vi "Keithley 2002 DCV Config.vi"(0 "GPIB address":string="16", 1 "range value (volts)":dbl=1000.0 min=0.2 max=1000.0 format="%^.2e", 2 "range (auto:0)":u16(ring) items=["autorange", "autorange once", "set min range", "set max range", "set range value"], 3 "dig. filter count":dbl=10.0 min=1.0 max=100.0 step=1.0 format="%^.2e", 4 "digital filter (off:0)":u16(ring) items=["off", "auto filter", "auto filter once", "moving filter", "repeating filter"], 5 "integration time (0:auto)":u16(ring) items=["automatic", "automatic once", "set to minimum", "set to maximum", "set aperature value", "set NPLC value"], 7 "integ. value":dbl=0.01667 format="%^.2e", 8 "advanced filter (off:0)":u16(ring) items=["off", "enabled"], 9 "resolution (4.5 digits:3)":u16(ring)=3 items=["auto resolution", "auto resolution once", "3.5 digits", "4.5 digits", "5.5 digits", "6.5 digits", "7.5 digits", "8.5 digits"], 10 "noise tolerance (%)":dbl=1.0 min=0.0 max=100.0 step=1.0 format="%^.2e", 11 "error in":T1, 12 "reference (off:0)":u16(ring) items=["off", "set reference value"], 13 "reference value (volts)":dbl min=-1100.0 max=1100.0 format="%^.2e") -> (15 "error out":T1)   [LabVIEW 2020]
doc: "This VI is used to configure the settings for the DC voltage measurements. The instrument can be in any mode when this VI is run. The settings will go into effect and the instrument will go into the DC voltage mode."
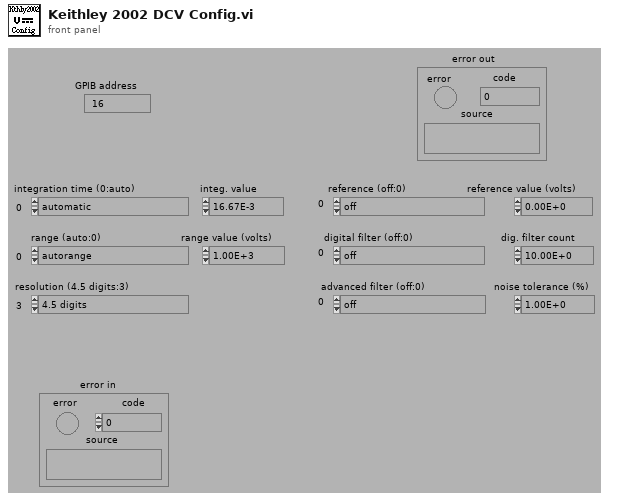
[diagram p1: front panel]
types:
  T1 = cluster{"error":bool, "code":i32, "source":string}
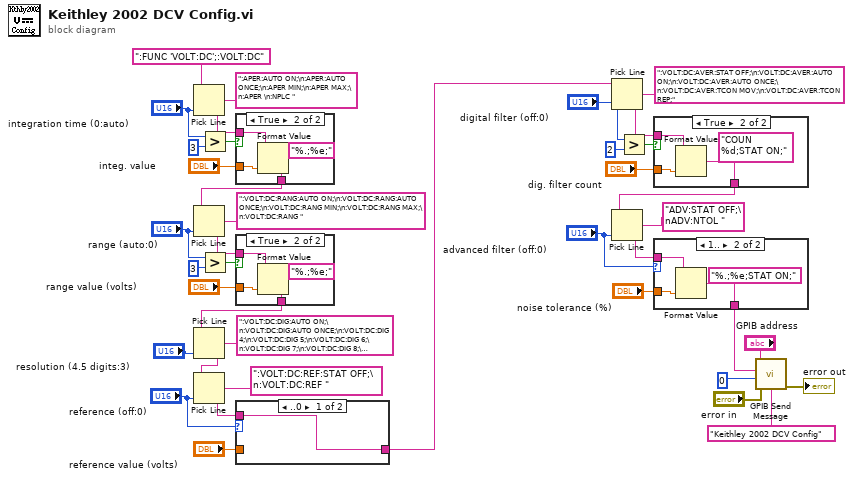
[diagram p0: block diagram]
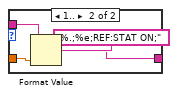
[diagram p4: hidden frame]
diagram:
  n1 = Pick Line(string ("")=":FUNC 'VOLT:DC';:VOLT:DC", multi-line string=":APER:AUTO ON;\n:APER:AUTO ONCE;\n:APER MIN;\n:APER MAX;\n:APER \n:NPLC ", line index="integration time (0:auto)") -> (output string=w34:string)
  n2 = Greater?(x="integration time (0:auto)", y=3) -> (0:w35:bool)
  n3 = Greater?(x="range (auto:0)", y=3) -> (0:w32:bool)
  n4 = case shown="True" w35 {
    tunnel: "integ. value" -> [_ w44]
    tunnel: w34 -> [w41 w43]
    tunnel: [w41 w42] -> w27
    frame False {
    }
    frame True {
      n5 = Format Value(string ("")=w43, format string="%.;%e;", value (0)=w44) -> (output string=w42:string)
    }
  }
  n6 = Pick Line(string ("")=w27, multi-line string=":VOLT:DC:RANG:AUTO ON;\n:VOLT:DC:RANG:AUTO ONCE;\n:VOLT:DC:RANG MIN;\n:VOLT:DC:RANG MAX;\n:VOLT:DC:RANG ", line index="range (auto:0)") -> (output string=w33:string)
  n7 = case shown="True" w32 {
    tunnel: "range value (volts)" -> [_ w49]
    tunnel: w33 -> [w46 w48]
    tunnel: [w46 w47] -> w24
    frame False {
    }
    frame True {
      n8 = Format Value(string ("")=w48, format string="%.;%e;", value (0)=w49) -> (output string=w47:string)
    }
  }
  n9 = Pick Line(string ("")=w24, multi-line string=":VOLT:DC:DIG:AUTO ON;\n:VOLT:DC:DIG:AUTO ONCE;\n:VOLT:DC:DIG 4;\n:VOLT:DC:DIG 5;\n:VOLT:DC:DIG 6;\n:VOLT:DC:DIG 7;\n:VOLT:DC:DIG 8;\n:Volt:DC:Dig 9;", line index="resolution (4.5 digits:3)") -> (output string=w20:string)
  n10 = Pick Line(string ("")=w20, multi-line string=":VOLT:DC:REF:STAT OFF;\n:VOLT:DC:REF ", line index="reference (off:0)") -> (output string=w23:string)
  n11 = case shown="..0" "reference (off:0)" {
    tunnel: "reference value (volts)" -> [_ w55]
    tunnel: w23 -> [w51 w54]
    tunnel: [w51 w52] -> w1
    frame ..0 {
    }
    frame 1.. {
      n12 = Format Value(string ("")=w54, format string="%.;%e;REF:STAT ON;", value (0)=w55) -> (output string=w52:string)
    }
  }
  n13 = Pick Line(string ("")=w1, multi-line string=":VOLT:DC:AVER:STAT OFF;\n:VOLT:DC:AVER:AUTO ON;\n:VOLT:DC:AVER:AUTO ONCE;\n:VOLT:DC:AVER:TCON MOV;\n:VOLT:DC:AVER:TCON REP;", line index="digital filter (off:0)") -> (output string=w17:string)
  n14 = Greater?(x="digital filter (off:0)", y=2) -> (0:w14:bool)
  n15 = case shown="True" w14 {
    tunnel: "dig. filter count" -> [_ w60]
    tunnel: w17 -> [w56 w59]
    tunnel: [w56 w58] -> w6
    frame False {
    }
    frame True {
      n16 = Format Value(string ("")=w59, format string="COUN %d;STAT ON;", value (0)=w60) -> (output string=w58:string)
    }
  }
  n17 = Pick Line(string ("")=w6, multi-line string="ADV:STAT OFF;\nADV:NTOL ", line index="advanced filter (off:0)") -> (output string=w10:string)
  n18 = case shown="1.." "advanced filter (off:0)" {
    tunnel: "noise tolerance (%)" -> [_ w65]
    tunnel: w10 -> [w61 w64]
    tunnel: [w61 w63] -> w7
    frame ..0 {
    }
    frame 1.. {
      n19 = Format Value(string ("")=w64, format string="%.;%e;STAT ON;", value (0)=w65) -> (output string=w63:string)
    }
  }
  n20 = call "GPIB Send Message.vi"("address string"="GPIB address", "write buffer"=w7, "source"="Keithley 2002 DCV Config", "write mode (set END:0)"=0, "error in"="error in") -> ("error out"=→"error out":T1)  [unwired: 2 in, 2 out]
